vi "Keithley 6514 Arm Layer Config.vi"(0 "Resource In":refnum<visa-resource-name>, 1 "Check For SCPI Errors? (T)":bool=TRUE, 2 "async trigger link input (line 1:1)":u16(ring)=1 items=["line 1", "line 1", "line 2", "line 3", "line 4", "line 5", "line 6"], 3 "Timer (0.1 secs)":dbl=0.1 min=0.0 max=99999.999 format="%.3f", 5 "count (set:0)":u16(ring) items=["set  value", "infinite", "min", "max"], 7 "count value (1)":i16=1 min=1 max=2500 step=1, 9 "direction":bool, 11 "error in (no error)":T1, 12 "output trigger":bool, 13 "async trigger link output (line 2:2)":u16(ring)=2 items=["line 1", "line 1", "line 2", "line 3", "line 4", "line 5", "line 6"], 14 "source (imm:1)":u16(ring) items=["immediate", "timer", "bus", "trigger link", "PSTEST", "NSTEST", "manual"]) -> (4 "Resource Out (dupl)":refnum<visa-resource-name>, 15 "error out":T1)   [LabVIEW 2009, in "Keithley 6514 LV 2009.lvlib"]
doc: "This VI is used to configure the settings for the Arm Layer (Trigger) of the trigger model. \n\ncount:\n0 = Set Value\n1 = Inifinite\n2 = min\n3 = max\n\nsource:\n0 = Immediate\n1 = Timer\n2 = Bus\n3 = Tlink\n4 = PSTEST\n5 = NSTEST\n6 = Manual\n\ndirection:\nFALSE= acceptor\nTRUE = source\n\nCount Value:\n1 to 2500\n\nTimer:\n0.001 to 99999.999 seconds\n\nOutput Trigger:\nFALSE = none\nTRUE = Trigger\n\nAsync Trigger Link Input:\n1 = Line 1\n2 = Line 2\n3 = Line 3\n4 = Line 4\n5 = Line 5\n6 = Line 6\n\nAsync Trigger Link Output:\n1 = Line 1\n2 = Line 2\n3 = Line 3\n4 = Line 4\n5 = Line 5\n6 = Line 6"
uses:
  Keithley 6514 LV 2009.lvlib
panel:
  # "trigger\nnone"
  # "source\nacceptor"
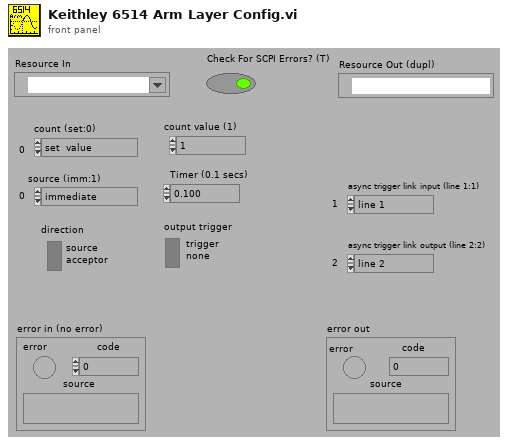
[diagram p1: front panel]
types:
  T1 = cluster{"error":bool, "code":i32, "source":string}
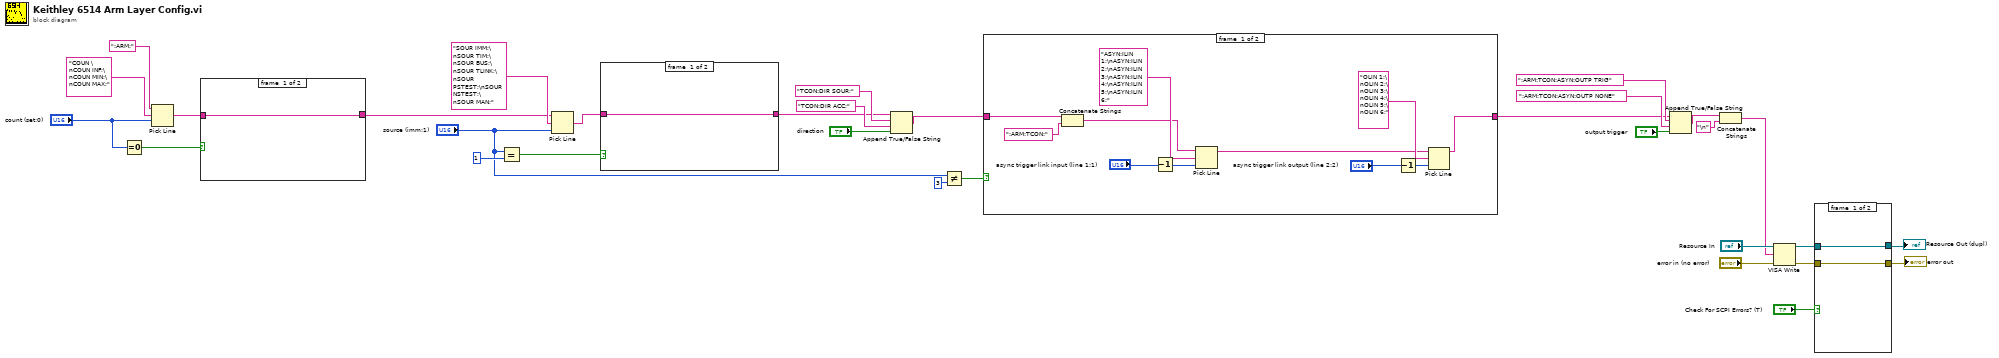
[diagram p0: block diagram]
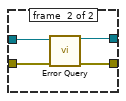
[diagram p2: hidden frame]
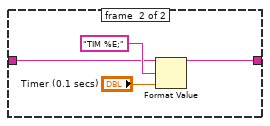
[diagram p3: hidden frame]
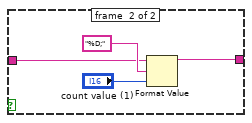
[diagram p5: hidden frame]
diagram:
  n1 = Equal To 0?(x="count (set:0)") -> (x = 0?=w30:bool)
  n2 = Pick Line(string ("")=":ARM:", multi-line string="COUN \nCOUN INF;\nCOUN MIN;\nCOUN MAX;", line index="count (set:0)") -> (output string=w18:string)
  n3 = case shown="True" w30 {
    tunnel: w18 -> [w33 w35]
    tunnel: [w33 w34] -> w17
    frame #0 {
    }
    frame #1 {
      n4 = Format Value(string ("")=w35, format string="%D;", value (0)="count value (1)") -> (output string=w34:string)
    }
  }
  n5 = Equal?(x="source (imm:1)", y=u16 1) -> (x = y?=w16:bool)
  n6 = Pick Line(string ("")=w17, multi-line string="SOUR IMM;\nSOUR TIM;\nSOUR BUS;\nSOUR TLINK;\nSOUR PSTEST;\nSOUR NSTEST;\nSOUR MAN;", line index="source (imm:1)") -> (output string=w15:string)
  n7 = case shown="True" w16 {
    tunnel: w15 -> [w38 w40]
    tunnel: [w38 w39] -> w14
    frame #0 {
    }
    frame #1 {
      n8 = Format Value(string ("")=w40, format string="TIM %E;", value (0)="Timer (0.1 secs)") -> (output string=w39:string)
    }
  }
  n9 = Append True/False String(1:"direction", 2:"TCON:DIR ACC;", 3:"TCON:DIR SOUR;", 4:w14) -> (0:w12:string)
  n10 = Not Equal?(x="source (imm:1)", y=u16 3) -> (x != y?=w13:bool)
  n11 = case shown="False" w13 {
    tunnel: w12 -> [w46 w54]
    tunnel: [w43 w54] -> w11
    frame #0 {
      n12 = Concatenate Strings(w46, ":ARM:TCON:") -> (w51:string)
      n13 = Decrement(x="async trigger link input (line 1:1)") -> (x-1=w48:u16)
      n14 = Pick Line(string ("")=w51, multi-line string="ASYN:ILIN 1;\nASYN:ILIN 2;\nASYN:ILIN 3;\nASYN:ILIN 4;\nASYN:ILIN 5;\nASYN:ILIN 6;", line index=w48) -> (output string=w44:string)
      n15 = Decrement(x="async trigger link output (line 2:2)") -> (x-1=w45:u16)
      n16 = Pick Line(string ("")=w44, multi-line string="OLIN 1;\nOLIN 2;\nOLIN 3;\nOLIN 4;\nOLIN 5;\nOLIN 6;", line index=w45) -> (output string=w43:string)
    }
    frame #1 {
    }
  }
  n17 = Append True/False String(1:"output trigger", 2:":ARM:TCON:ASYN:OUTP NONE", 3:":ARM:TCON:ASYN:OUTP TRIG", 4:w11) -> (0:w10:string)
  n18 = Concatenate Strings(w10, "\n") -> (w7:string)
  n19 = VISA Write(VISA resource name="Resource In", write buffer=w7, error in (no error)="error in (no error)") -> (VISA resource name out=w4:refnum<visa-resource-name>, error out=w3:errorcluster)  [unwired: 1 out]
  n20 = case shown="True" "Check For SCPI Errors? (T)" {
    tunnel: w4 -> [w56 w60]
    tunnel: w3 -> [w55 w59]
    tunnel: [w56 w58] -> w2
    tunnel: [w55 w57] -> w1
    frame #0 {
    }
    frame #1 {
      n21 = call "Error Query.vi"("VISA Resource In"=w60, "error in (no error)"=w59) -> ("VISA Resource Out (dupl)"=w58:refnum<visa-resource-name>, "error out"=w57:errorcluster)  [unwired: 10 in, 2 out]
    }
  }
  "error out" <- w1
  "Resource Out (dupl)" <- w2
